vi "InitCSMs.vi"(7 "Enable building lvlibp?":bool, 8 "error in (no error)":errorcluster, 11 "testcase-CSMSyncMessage in":refnum<class "testcase-CSMMessage.lvclass">) -> (0 "error out":errorcluster, 3 "testcase-CSMSyncMessage out":refnum<class "testcase-CSMMessage.lvclass">)   [LabVIEW 2017, in "testcase-CSMMessage.lvclass"]
uses:
  testcase-CSMMessage.lvclass
  testcase-CSMMessage.lvclass/testcase-CSMMessage.ctl
  CSM/Normal-CSM.vi
  CSM/Chain1.vi
  CSM/Chain2.vi
  CSM/Chain3.vi
  <vilib>/AppBuilder/AB_API_Simple/Build (path).vi
  CSM/CSM-Testcase.lvlib
  src/user.lib/_NEVSTOP/Communicable State Machine(CSM)/Communicable State Machine.lvlib
  <vilib>/AppBuilder/AB_API_Simple/NI_App_Builder_API.lvlib
panel:
  out "Waited (ms)":u32
  out "CSMs Left":string[](array[string])
  out "Generated files":path[](array[path])
  out "CSMs":string[](array[string])
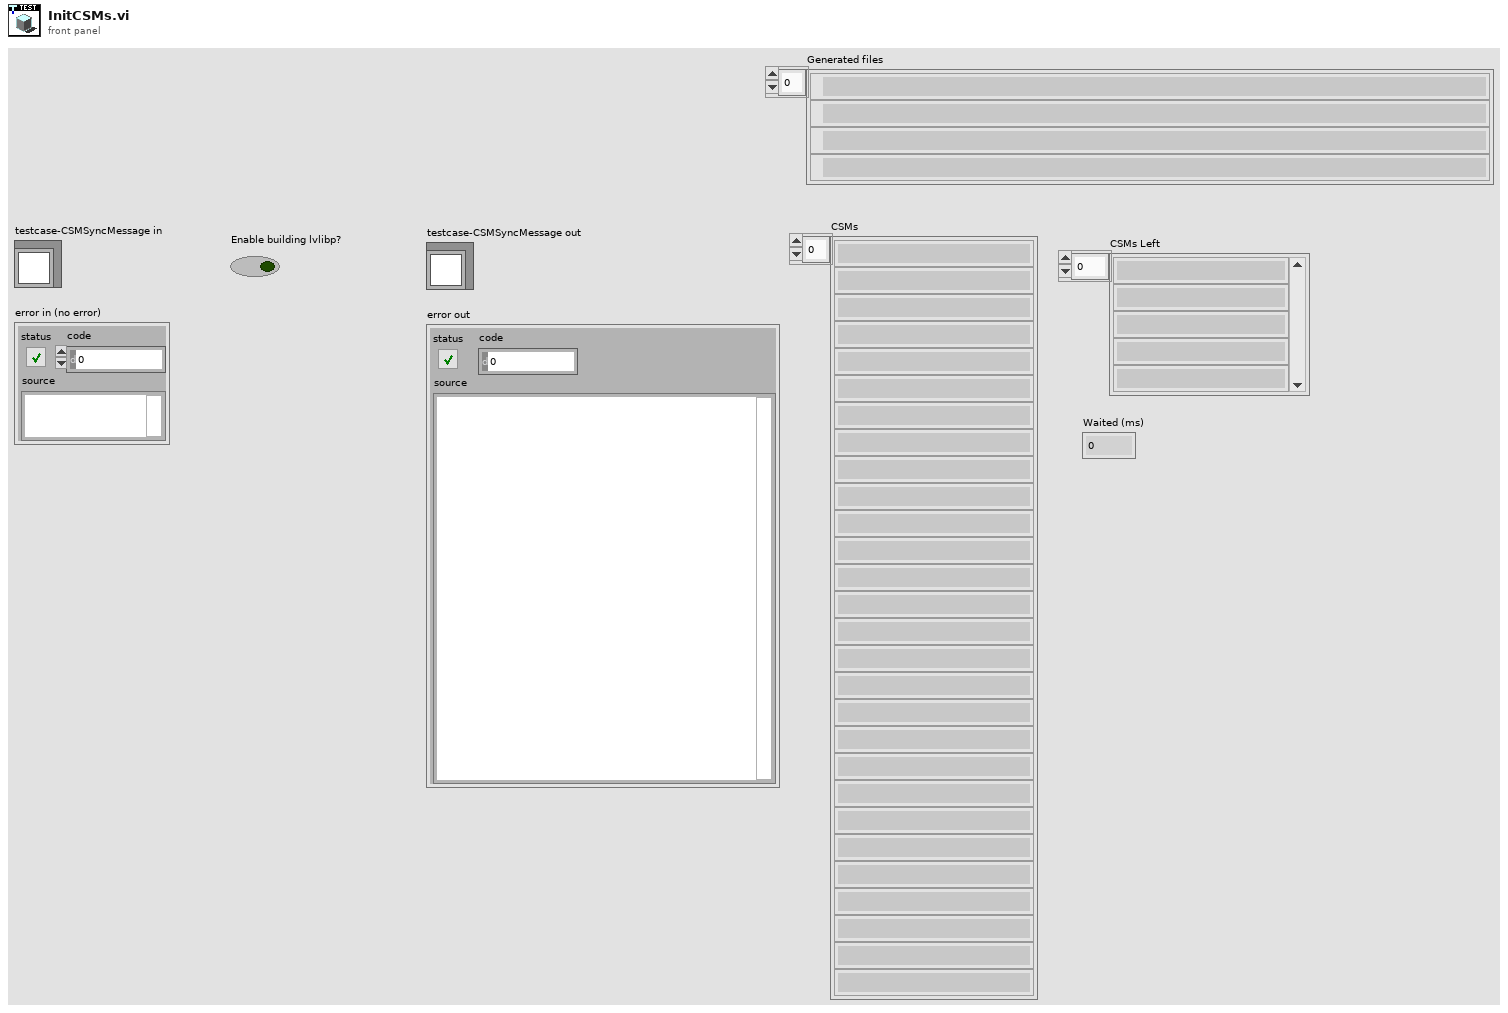
[diagram p1: front panel]
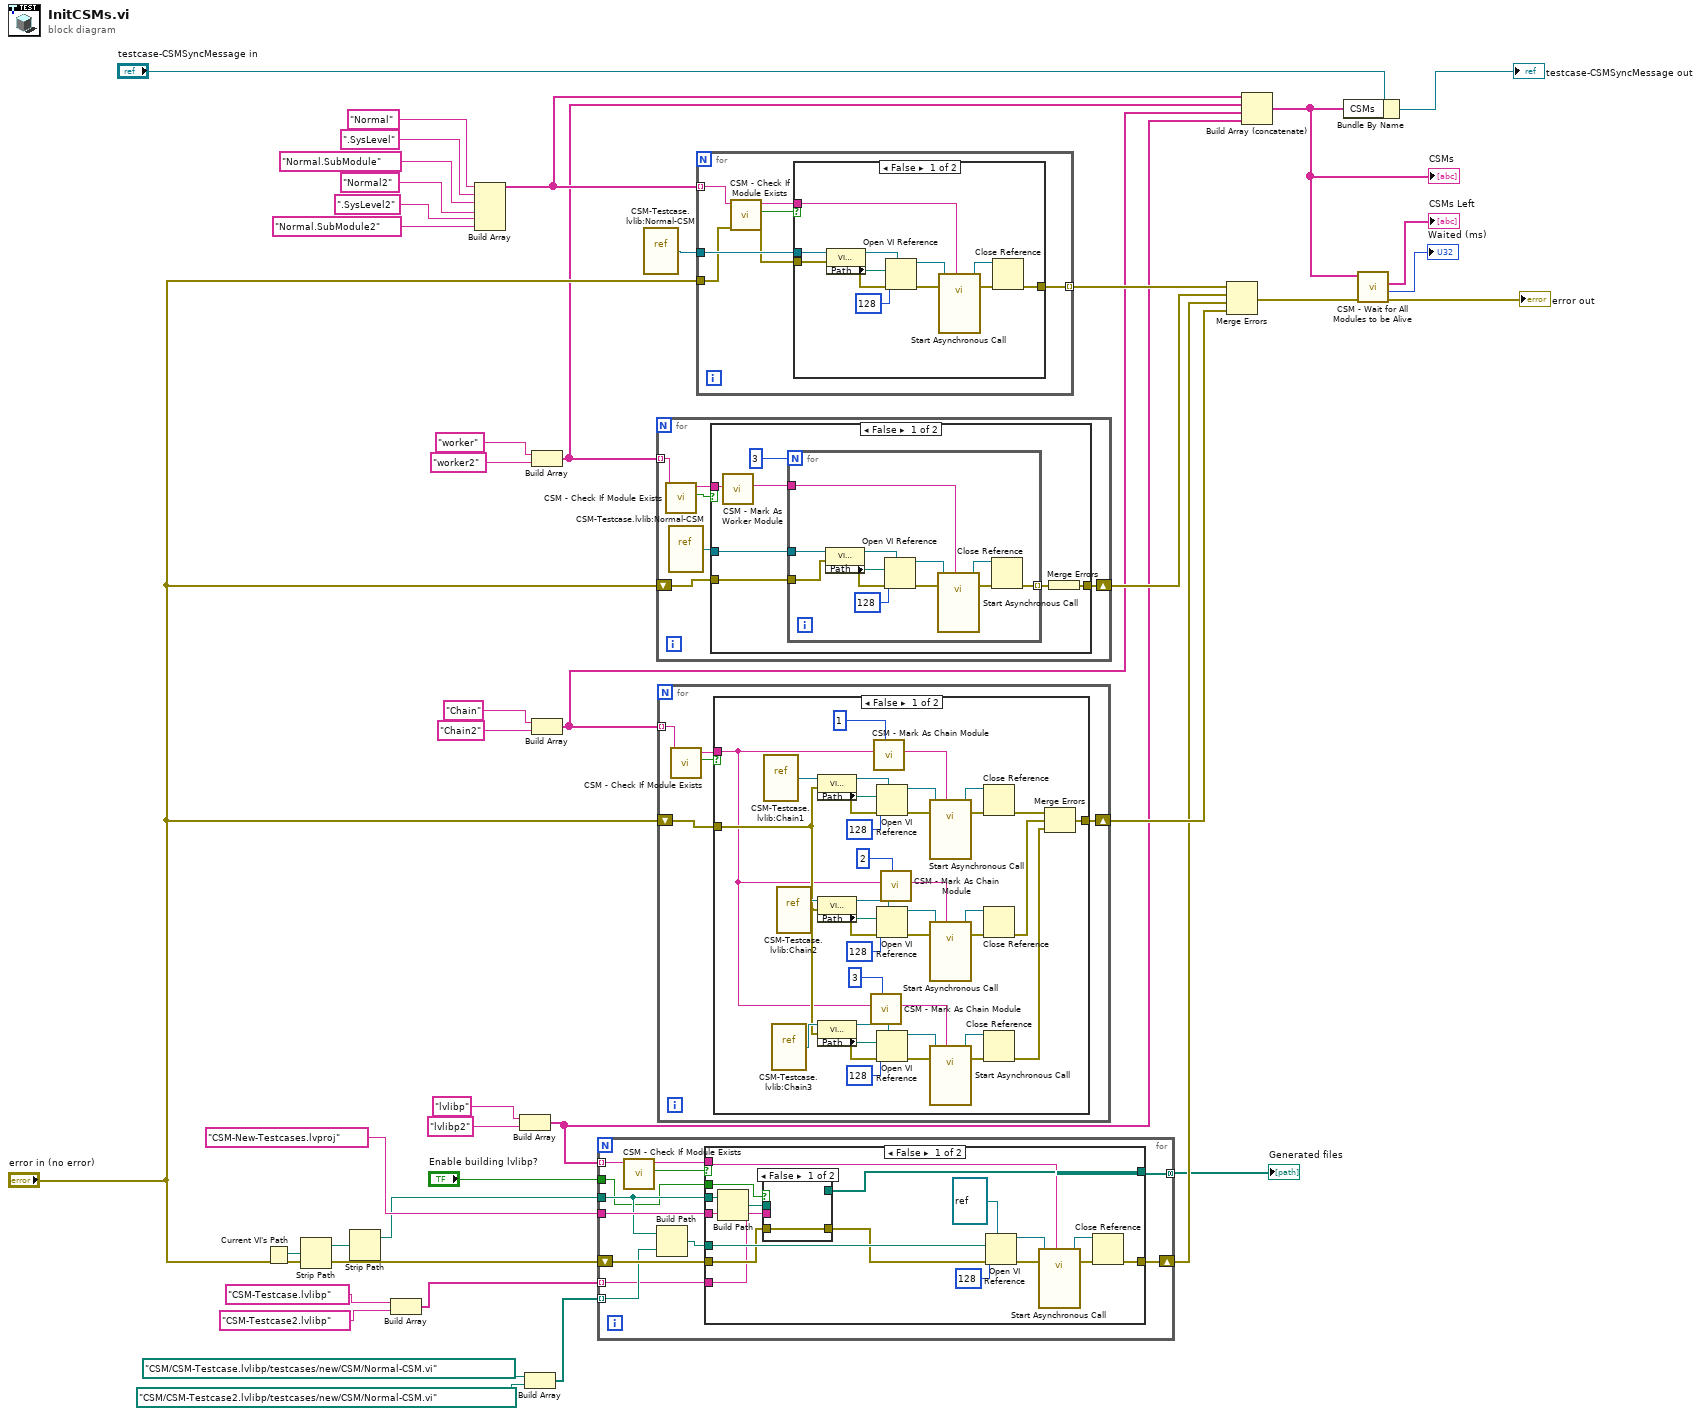
[diagram p0: block diagram]
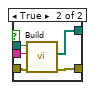
[diagram p2: hidden frame]
diagram:
  n1 = Current VI's Path() -> (path=w36:path)
  n2 = Strip Path(path=w36) -> (stripped path=w37:path)  [unwired: 1 out]
  n3 = Strip Path(path=w37) -> (stripped path=w38:path)  [unwired: 1 out]
  n4 = Build Array("CSM-Testcase.lvlibp" ("Name of build specification (if empty: build all)"), "CSM-Testcase2.lvlibp" ("Name of build specification (if empty: build all)")) -> (w8:string[])
  n5 = Build Array("Normal" ("Name (\"\" to Use UUID)"), ".SysLevel" ("Name (\"\" to Use UUID)"), "Normal.SubModule" ("Name (\"\" to Use UUID)"), "Normal2" ("Name (\"\" to Use UUID)"), ".SysLevel2" ("Name (\"\" to Use UUID)"), "Normal.SubModule2" ("Name (\"\" to Use UUID)")) -> (w32:string[])
  n6 = Build Array("lvlibp" ("Name (\"\" to Use UUID)"), "lvlibp2" ("Name (\"\" to Use UUID)")) -> (w14:string[])
  n7 = Build Array(path "CSM/CSM-Testcase.lvlibp/testcases/new/CSM/Normal-CSM.vi" ("vi path"), path "CSM/CSM-Testcase2.lvlibp/testcases/new/CSM/Normal-CSM.vi" ("vi path")) -> (w11:path[])
  n8 = Build Array("worker" ("Name (\"\" to Use UUID)"), "worker2" ("Name (\"\" to Use UUID)")) -> (w20:string[])
  n9 = Build Array("Chain" ("Name (\"\" to Use UUID)"), "Chain2" ("Name (\"\" to Use UUID)")) -> (w17:string[])
  n10 = for {
    tunnel: "CSM-New-Testcases.lvproj" ("name or relative path") -> [w51]
    tunnel: w38 -> [w46]
    shift-right: [w50] -> w35
    shift-left: "error in (no error)" -> [w52]
    tunnel: w14 -> [w48] mode=indexing
    tunnel: w11 -> [w47] mode=indexing
    tunnel: w8 -> [w44] mode=indexing
    tunnel: [w43] -> w7 mode=concatenating
    tunnel: "Enable building lvlibp?" -> [w42]
    n11 = call "CSM - Check If Module Exists.vi"("CSM Name"=w48) -> ("Exist?"=w53:bool, "CSM Name (Dup)"=w49:string)  [unwired: 8 in, 1 out]
    n12 = Build Path(base path=w46, name or relative path=w47) -> (appended path=w45:path)
    n13 = case shown="False" w53 {
      tunnel: [w70 w77] -> w50
      tunnel: w45 -> [w63 _]
      tunnel: w46 -> [w62 _]
      tunnel: w51 -> [w60 _]
      tunnel: w49 -> [w59 _]
      tunnel: w52 -> [w58 w77]
      tunnel: w44 -> [w56 _]
      tunnel: [w55 _] -> w43
      tunnel: w42 -> [w54 _]
      frame False {
        n14 = Build Path(base path=w62, name or relative path=w60) -> (appended path=w61:path)
        n15 = case shown="False" w54 {
          tunnel: w61 -> [_ w76]
          tunnel: w58 -> [w71 w75]
          tunnel: [w71 w74] -> w57
          tunnel: w56 -> [_ w73]
          tunnel: [_ w72] -> w55
          frame False {
          }
          frame True {
            n16 = call-poly <vilib>:"Build.vi"("error in (no error)"=w75, "Name of build specification (if empty: build all)"=w73, "Path to project"=w76) -> ("error out"=w74:errorcluster, "Generated files"=w72:path[])  [unwired: 7 in]
          }
        }
        n17 = Open VI Reference(type specifier VI Refnum (for type only)=refnum<vi> refnum ("reference out"), vi path=w63, options=128, error in (no error)=w57) -> (vi reference=w66:refnum<vi>, error out=w68:errorcluster)  [unwired: 2 in]
        n18 = call-by-ref "Start Asynchronous Call"(reference=w66, error in=w68, "Name (\"\" to Use UUID)"=w59) -> (reference out=w65:refnum<vi>, error out=w67:errorcluster)  [unwired: 11 in]
        n19 = Close Reference(reference=w65, error in (no error)=w67) -> (error out=w70:errorcluster)
      }
      frame True {
      }
    }
  }
  "Generated files" <- w7
  n20 = vi-ref "CSM-Testcase.lvlib:Normal-CSM.vi"() -> (w28:refnum<vi>)
  n21 = for {
    shift-right: [w80] -> w34
    shift-left: "error in (no error)" -> [w83]
    tunnel: w20 -> [w79] mode=indexing
    n22 = call "CSM - Check If Module Exists.vi"("CSM Name"=w79) -> ("Exist?"=w82:bool, "CSM Name (Dup)"=w81:string)  [unwired: 8 in, 1 out]
    n23 = vi-ref "CSM-Testcase.lvlib:Normal-CSM.vi"() -> (w78:refnum<vi>)
    n24 = case shown="False" w82 {
      tunnel: w78 -> [w90 _]
      tunnel: [w84 w103] -> w80
      tunnel: w83 -> [w86 w103]
      tunnel: w81 -> [w85 _]
      frame False {
        n25 = call "CSM - Mark As Worker Module.vi"("CSM Name"=w85) -> ("CSM Name (Marked As Worker)"=w87:string)  [unwired: 9 in]
        n26 = for {
          N: 3 -> [_]
          tunnel: w90 -> [w94]
          tunnel: w87 -> [w93]
          tunnel: [w92] -> w88 mode=indexing
          tunnel: w86 -> [w91]
          n27 = property class="VI (strict)"(reference=w94, error in=w91) -> (reference out=w100:refnum<vi>, error out=w98:errorcluster, "Path"=w97:path)
          n28 = Open VI Reference(type specifier VI Refnum (for type only)=w100, vi path=w97, options=128, error in (no error)=w98) -> (vi reference=w96:refnum<vi>, error out=w101:errorcluster)  [unwired: 2 in]
          n29 = call-by-ref "Start Asynchronous Call"(reference=w96, error in=w101, "Name (\"\" to Use UUID)"=w93) -> (reference out=w95:refnum<vi>, error out=w99:errorcluster)  [unwired: 11 in]
          n30 = Close Reference(reference=w95, error in (no error)=w99) -> (error out=w92:errorcluster)
        }
        n31 = Merge Errors(w88) -> (w84:errorcluster)
      }
      frame True {
      }
    }
  }
  n32 = for {
    shift-right: [w106] -> w40
    shift-left: "error in (no error)" -> [w108]
    tunnel: w17 -> [w104] mode=indexing
    n33 = call "CSM - Check If Module Exists.vi"("CSM Name"=w104) -> ("Exist?"=w107:bool, "CSM Name (Dup)"=w105:string)  [unwired: 8 in, 1 out]
    n34 = case shown="False" w107 {
      tunnel: [w111 w148] -> w106
      tunnel: w108 -> [w110 w148]
      tunnel: w105 -> [w109 _]
      frame False {
        n35 = vi-ref "CSM-Testcase.lvlib:Chain1.vi"() -> (w147:refnum<vi>)
        n36 = vi-ref "CSM-Testcase.lvlib:Chain3.vi"() -> (w129:refnum<vi>)
        n37 = vi-ref "CSM-Testcase.lvlib:Chain2.vi"() -> (w130:refnum<vi>)
        n38 = property class="VI (strict)"(reference=w147, error in=w110) -> (reference out=w144:refnum<vi>, error out=w142:errorcluster, "Path"=w141:path)
        n39 = property class="VI (strict)"(reference=w130, error in=w110) -> (reference out=w133:refnum<vi>, error out=w135:errorcluster, "Path"=w136:path)
        n40 = property class="VI (strict)"(reference=w129, error in=w110) -> (reference out=w126:refnum<vi>, error out=w124:errorcluster, "Path"=w123:path)
        n41 = call "CSM - Mark As Chain Module.vi"("Order"=3, "CSM Name"=w109) -> ("CSM Name (Marked As Chain)"=w117:string)  [unwired: 8 in]
        n42 = call "CSM - Mark As Chain Module.vi"("Order"=1, "CSM Name"=w109) -> ("CSM Name (Marked As Chain)"=w115:string)  [unwired: 8 in]
        n43 = Open VI Reference(type specifier VI Refnum (for type only)=w144, vi path=w141, options=128, error in (no error)=w142) -> (vi reference=w140:refnum<vi>, error out=w145:errorcluster)  [unwired: 2 in]
        n44 = Open VI Reference(type specifier VI Refnum (for type only)=w133, vi path=w136, options=128, error in (no error)=w135) -> (vi reference=w137:refnum<vi>, error out=w132:errorcluster)  [unwired: 2 in]
        n45 = Open VI Reference(type specifier VI Refnum (for type only)=w126, vi path=w123, options=128, error in (no error)=w124) -> (vi reference=w122:refnum<vi>, error out=w127:errorcluster)  [unwired: 2 in]
        n46 = call "CSM - Mark As Chain Module.vi"("Order"=2, "CSM Name"=w109) -> ("CSM Name (Marked As Chain)"=w116:string)  [unwired: 8 in]
        n47 = call-by-ref "Start Asynchronous Call"(reference=w140, error in=w145, "Name (\"\" to Use UUID)"=w115) -> (reference out=w139:refnum<vi>, error out=w143:errorcluster)  [unwired: 11 in]
        n48 = call-by-ref "Start Asynchronous Call"(reference=w137, error in=w132, "Name (\"\" to Use UUID)"=w116) -> (reference out=w138:refnum<vi>, error out=w134:errorcluster)  [unwired: 11 in]
        n49 = call-by-ref "Start Asynchronous Call"(reference=w122, error in=w127, "Name (\"\" to Use UUID)"=w117) -> (reference out=w121:refnum<vi>, error out=w125:errorcluster)  [unwired: 11 in]
        n50 = Close Reference(reference=w139, error in (no error)=w143) -> (error out=w120:errorcluster)
        n51 = Close Reference(reference=w138, error in (no error)=w134) -> (error out=w119:errorcluster)
        n52 = Close Reference(reference=w121, error in (no error)=w125) -> (error out=w118:errorcluster)
        n53 = Merge Errors(w120, w119, w118) -> (w111:errorcluster)
      }
      frame True {
      }
    }
  }
  n54 = for {
    tunnel: w28 -> [w155]
    tunnel: w32 -> [w151] mode=indexing
    tunnel: [w154] -> w33 mode=indexing
    tunnel: "error in (no error)" -> [w153]
    n55 = call "CSM - Check If Module Exists.vi"("Error In"=w153, "CSM Name"=w151) -> ("error out"=w152:errorcluster, "Exist?"=w149:bool, "CSM Name (Dup)"=w150:string)  [unwired: 7 in]
    n56 = case shown="False" w149 {
      tunnel: w155 -> [w159 _]
      tunnel: [w158 w168] -> w154
      tunnel: w152 -> [w157 w168]
      tunnel: w150 -> [w156 _]
      frame False {
        n57 = property class="VI (strict)"(reference=w159, error in=w157) -> (reference out=w165:refnum<vi>, error out=w163:errorcluster, "Path"=w162:path)
        n58 = Open VI Reference(type specifier VI Refnum (for type only)=w165, vi path=w162, options=128, error in (no error)=w163) -> (vi reference=w161:refnum<vi>, error out=w166:errorcluster)  [unwired: 2 in]
        n59 = call-by-ref "Start Asynchronous Call"(reference=w161, error in=w166, "Name (\"\" to Use UUID)"=w156) -> (reference out=w160:refnum<vi>, error out=w164:errorcluster)  [unwired: 11 in]
        n60 = Close Reference(reference=w160, error in (no error)=w164) -> (error out=w158:errorcluster)
      }
      frame True {
      }
    }
  }
  n61 = Merge Errors(w33, w34, w35, w40) -> (w6:errorcluster)
  n62 = Build Array (concatenate)(w32, w20, w17, w14) -> (w4:string[])
  "CSMs" <- w4
  n63 = Bundle By Name(cluster="testcase-CSMSyncMessage in", "CSMs"=w4) -> (→"testcase-CSMSyncMessage out":refnum<class "testcase-CSMMessage.lvclass">)
  n64 = call "CSM - Wait for All Modules to be Alive.vi"("Error In"=w6, "CSM Names"=w4) -> ("error out"=→"error out":errorcluster, "Waited (ms)"=→"Waited (ms)":u32, "CSMs Left"=→"CSMs Left":string[])  [unwired: 7 in]
